vi "Get Server State Ref.vi"(11 "Template Server in":refnum<class "HVC6.lvclass">) -> (2 "Server State Ref":refnum<data-value>, 3 "Template Server out":refnum<class "HVC6.lvclass">)   [LabVIEW 2019, in "HVC6.lvlib" / "HVC6.lvclass"]
uses:
  HVC6.lvclass
  typeDefs/Server State Data.ctl
  HVC6.lvclass/HVC6.ctl
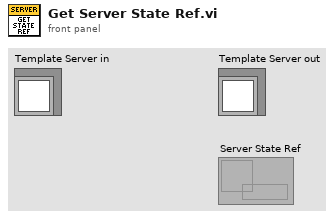
[diagram p1: front panel]
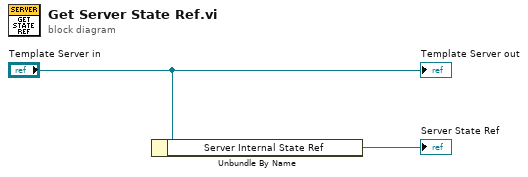
[diagram p0: block diagram]
diagram:
  n1 = Unbundle By Name("Template Server in") -> ("Server Internal State Ref"=→"Server State Ref":refnum<data-value>)
  "Template Server out" <- "Template Server in"
